vi "CSM - List Log Filter Rules As Strings.vi"(8 "Error In":errorcluster caption="error in (no error)") -> (0 "error out":errorcluster, 2 "Rule Strings":string[](array[string]))   [LabVIEW 2017, in "Communicable State Machine.lvlib"]
doc: "Lists global filter rules in string format, with each rule occupying one line for user viewing. This VI is primarily used for background log file saving, debugging interface viewing, and so on.\n\n\n> [!NOTE] <b>Global Log Filter Rules</b>\n>\n> Global log filter rules allow a category of logs to be filtered out so they do not appear in the global log.\n>\n> The following are the three types of log filter rules:\n> - <b>Global Rules</b>: Apply to all modules meeting the conditions. You can configure the following settings:\n> - <b>Module Name</b>: All names of the module will be filtered.\n> - <b>Log Type</b>: Such as state, message, broadcast, module Initialization, and so on.\n> - <b>State Name</b>: Any module with the state name will be filtered.\n> - <b>State Type</b>: Type of state, such as internal state, external message, and so on.\n> - <b>Broadcast</b>: Broadcasts with the specified broadcast name will be filtered. Applies to Status Broadcast and Interrupt Broadcast logs.\n> - <b>User Log</b>: User logs with the specified user log name will be filtered.\n> - <b>Module Rules</b>: Apply to specific modules. You can configure the following settings:\n> - <b>Module Log Type</b>: Modules with the specified log types of the module are filtered.\n> - <b>State Name</b>: Modules with the specified state name are filtered.\n> - <b>State Type</b>: Modules with the specified state type are filtered.\n> - <b>Broadcast</b>: Modules with the specified broadcast name are filtered.\n> - <b>User Log</b>: Modules with the specified user log name are filtered.\n> - <b>Periodic Filter Rules</b>: This rule is currently only effective at the registration point because it is difficult to count numbers at the publication location.\n> - Whether to enable periodic filtering.\n> - <b>Threshold (#/s)</b>: Periodic filtering threshold.\n> - <b>CheckPeriod (s)</b>: Check window time.\n\n\n-- <b>Indicators</b> --\n- <b>Rule Strings</b>: Filter rule strings."
uses:
  Communicable State Machine.lvlib
  _Support/ChangeFlag/ChangeFlag-Read.vi
  _Support/ChangeFlag/ChangeFlagDB.vi
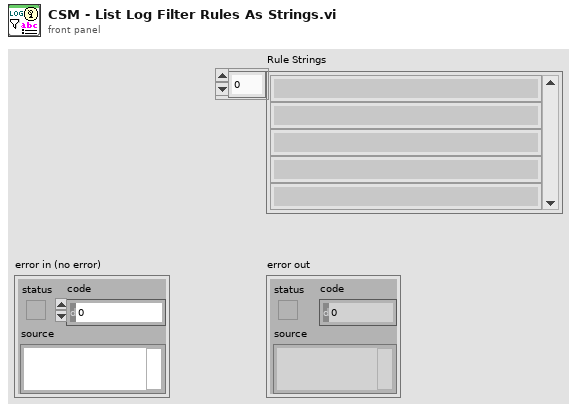
[diagram p1: front panel]
types:
  T1 = typedef "Communicable State Machine.lvlib/_CSM_GlobalLog Filter Rules - v1.2.ctl" = cluster{"Global":cluster{"CSM":string[], "LogType":T2[], "State":string[], "StateType":T3[], "Broadcast":string[], "UserLog":string[]}, "CSM":cluster{"LogType":cluster{"CSM":string, "LogType":T2}[], "State":cluster{"CSM":string, "State":string}[], "StateType":cluster{"CSM":string, "LogType":T3}[], "Broadcast":cluster{"CSM":string, "Broadcast":string}[], "UserLog":cluster{"CSM":string, "UserLog":string}[]}, "PeriodicMessageFilter":cluster{"Enable":bool, "Threshold(#/s)":dbl, "CheckPeriod(s)":dbl}}
  T2 = typedef "Communicable State Machine.lvlib/_CSM_GlobalLog_MSG_TYPE.ctl" = enum16{"User Log", "State Change", "Status", "Interrupt", "Register", "Unregister", "Error Log", "Module Created", "Module Destroyed", "Async Message", "No-Rep Async Message", "Sync Message", "AsyncMsg Complete", "SyncMsg Complete"}
  T3 = typedef "Communicable State Machine.lvlib/_CSM_GlobalLog_STATE_TYPE.ctl" = enum16{"State - Internal State", "State - External Message", "State - Response", "State - Complete"}
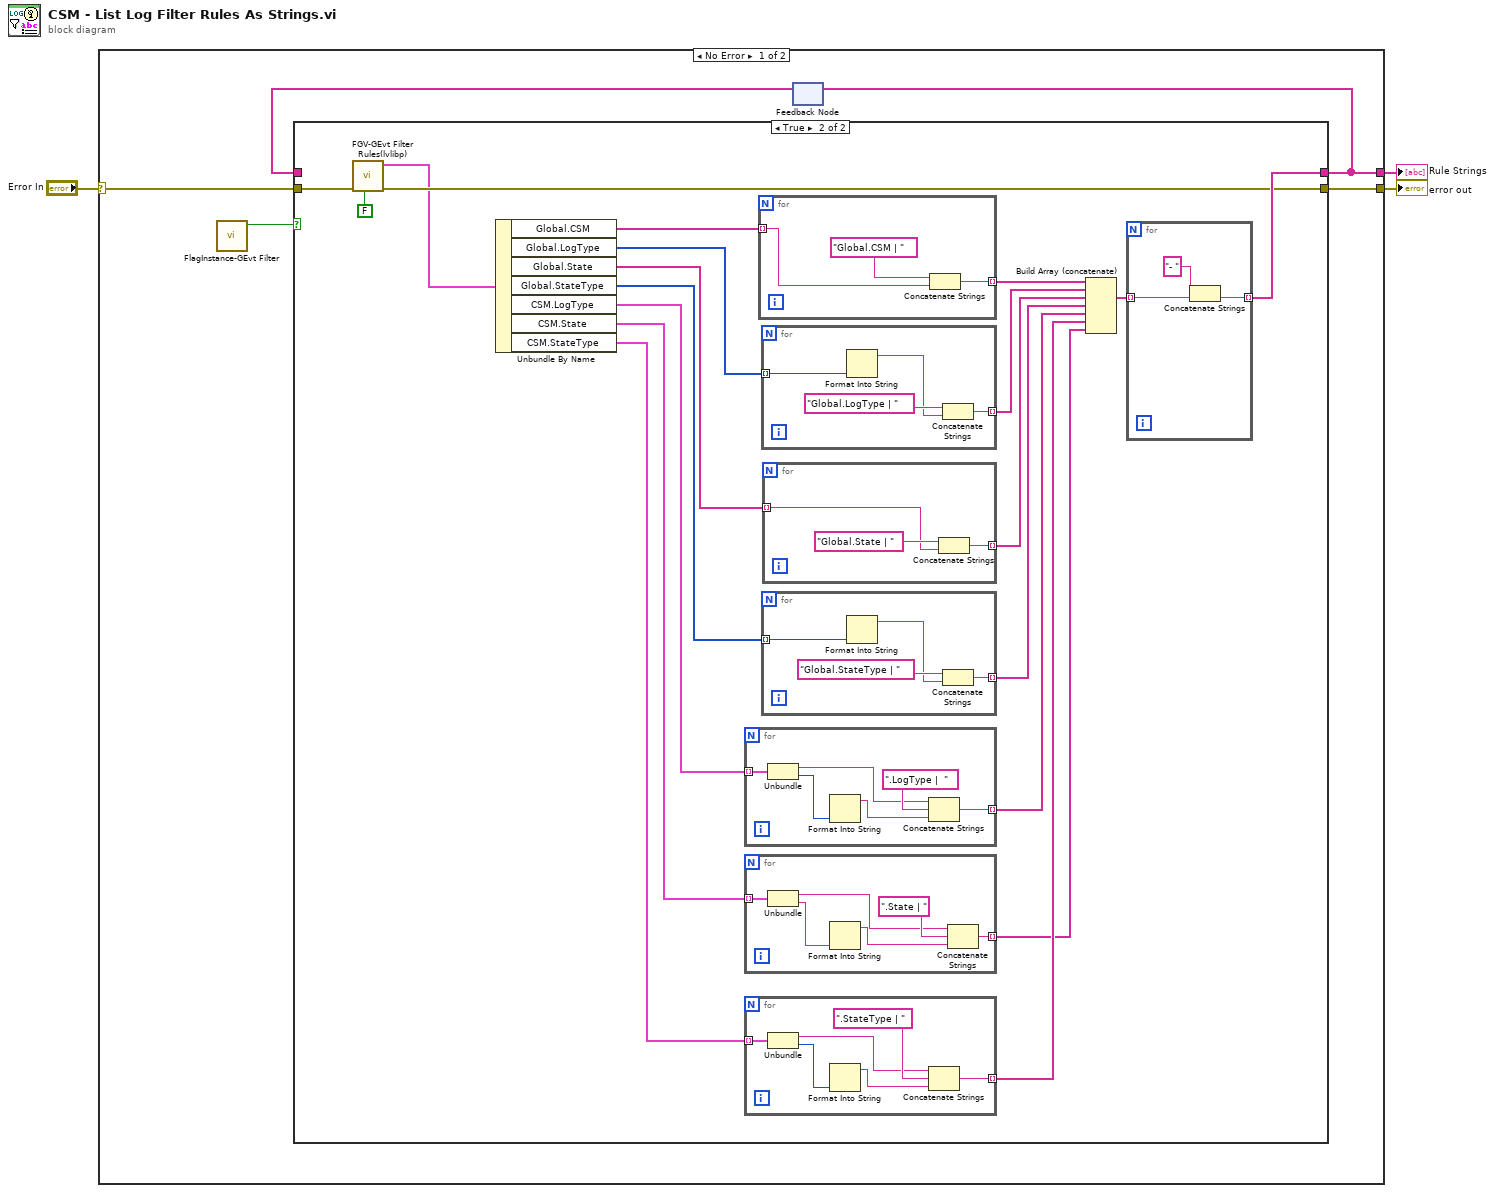
[diagram p0: block diagram]
diagram:
  n1 = case shown="No Error" "Error In" {
    selector: "Error In" -> [w8 w66]
    tunnel: [w7 w66] -> w2
    tunnel: [w5 _] -> w1
    frame No Error {
      n2 = call "FlagInstance-GEvt Filter.vi"() -> ("Changed"=w6:bool)  [unwired: 10 in, 1 out]
      n3 = feedback #1() -> (w4:string[])  [unwired: 1 in]
      n4 = case shown="True" w6 {
        tunnel: w8 -> [w9 w29]
        tunnel: [w10 w28] -> w5
        tunnel: [w9 w12] -> w7
        tunnel: w4 -> [w10 _]
        frame False {
        }
        frame True {
          n5 = call "FGV-GEvt Filter Rules(lvlibp).vi"("Set? (T)/Get(F)"=FALSE ("Set(T)/Get(F)"), "Error In"=w29) -> ("error out"=w12:errorcluster, "Rules-v1.2 out"=w11:T1)  [unwired: 8 in]
          n6 = Unbundle By Name(w11) -> ("Global.CSM"=w13:string[], "Global.LogType"=w15:T2[], "Global.State"=w17:string[], "Global.StateType"=w24:T3[], "CSM.LogType"=w19:cluster{"CSM":string, "LogType":T2}[], "CSM.State"=w21:cluster{"CSM":string, "State":string}[], "CSM.StateType"=w26:cluster{"CSM":string, "LogType":T3}[])
          n7 = for {
            tunnel: w19 -> [w53] mode=indexing
            tunnel: [w54] -> w20 mode=indexing
            n8 = Unbundle(w53) -> ("CSM"=w52:string, "LogType"=w51:T2)
            n9 = Format Into String(w51) -> (resulting string=w50:string)  [unwired: 3 in, 1 out]
            n10 = Concatenate Strings(w52, ".LogType |  " ("string"), w50) -> (w54:string)
          }
          n11 = for {
            tunnel: w21 -> [w47] mode=indexing
            tunnel: [w48] -> w22 mode=indexing
            n12 = Unbundle(w47) -> ("CSM"=w46:string, "State"=w45:string)
            n13 = Format Into String(w45) -> (resulting string=w44:string)  [unwired: 3 in, 1 out]
            n14 = Concatenate Strings(w46, ".State | " ("string"), w44) -> (w48:string)
          }
          n15 = for {
            tunnel: w26 -> [w34] mode=indexing
            tunnel: [w35] -> w27 mode=indexing
            n16 = Unbundle(w34) -> ("CSM"=w33:string, "LogType"=w32:T3)
            n17 = Format Into String(w32) -> (resulting string=w31:string)  [unwired: 3 in, 1 out]
            n18 = Concatenate Strings(w33, ".StateType | " ("string"), w31) -> (w35:string)
          }
          n19 = for {
            tunnel: w13 -> [w64] mode=indexing
            tunnel: [w63] -> w14 mode=indexing
            n20 = Concatenate Strings("Global.CSM | " ("string"), w64) -> (w63:string)
          }
          n21 = for {
            tunnel: w15 -> [w60] mode=indexing
            tunnel: [w61] -> w16 mode=indexing
            n22 = Format Into String(w60) -> (resulting string=w59:string)  [unwired: 3 in, 1 out]
            n23 = Concatenate Strings("Global.LogType | " ("string"), w59) -> (w61:string)
          }
          n24 = for {
            tunnel: w24 -> [w37] mode=indexing
            tunnel: [w39] -> w25 mode=indexing
            n25 = Format Into String(w37) -> (resulting string=w38:string)  [unwired: 3 in, 1 out]
            n26 = Concatenate Strings("Global.StateType | " ("string"), w38) -> (w39:string)
          }
          n27 = for {
            tunnel: w17 -> [w56] mode=indexing
            tunnel: [w57] -> w18 mode=indexing
            n28 = Concatenate Strings("Global.State | " ("string"), w56) -> (w57:string)
          }
          n29 = Build Array (concatenate)(w14, w16, w18, w25, w20, w27, w22) -> (w23:string[])
          n30 = for {
            tunnel: [w41] -> w28 mode=indexing
            tunnel: w23 -> [w42] mode=indexing
            n31 = Concatenate Strings("- " ("string"), w42) -> (w41:string)
          }
        }
      }
      n32 = feedback-in #1(w5) -> ()
    }
    frame Error {
    }
  }
  "error out" <- w2
  "Rule Strings" <- w1
